vi "test_harness_distance_between_points_squared.vi"() -> ()   [LabVIEW 2009]
panel:
  out "x = y?":bool
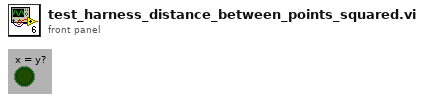
[diagram p1: front panel]
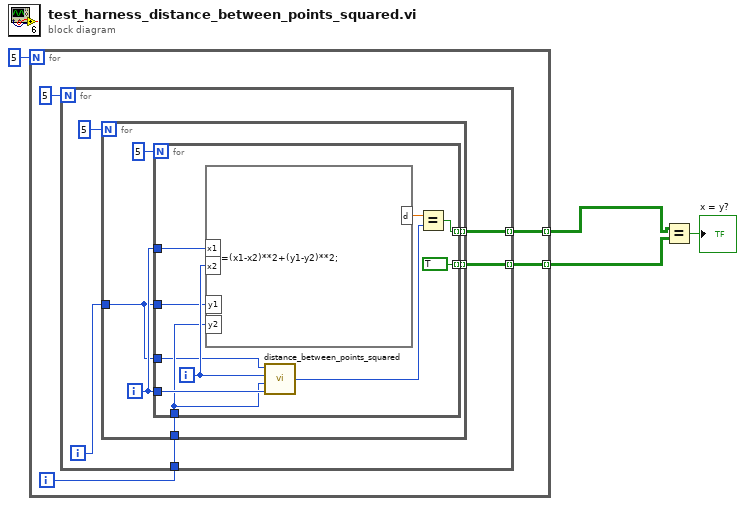
[diagram p0: block diagram]
diagram:
  n1 = for {
    N: 5 -> [_]
    tunnel: [w6] -> w3 mode=indexing
    tunnel: [w5] -> w2 mode=indexing
    i -> [w8]
    n2 = for {
      N: 5 -> [_]
      tunnel: w8 -> [w11]
      tunnel: [w10] -> w6 mode=indexing
      tunnel: [w9] -> w5 mode=indexing
      i -> [w12]
      n3 = for {
        N: 5 -> [_]
        tunnel: w12 -> [w17]
        tunnel: w11 -> [w18]
        tunnel: [w15] -> w10 mode=indexing
        tunnel: [w14] -> w9 mode=indexing
        i -> [w19]
        n4 = for {
          N: 5 -> [_]
          tunnel: w19 -> [w29]
          tunnel: w19 -> [w26]
          tunnel: w17 -> [w24]
          tunnel: w18 -> [w23]
          tunnel: w17 -> [w22]
          tunnel: [w21] -> w15 mode=indexing
          tunnel: [TRUE] -> w14 mode=indexing
          i -> [w25]
          n5 = formula code="d=(x1-x2)**2+(y1-y2)**2;"("x1"=w29, "x2"=w25, "y1"=w24, "y2"=w23) -> ("d"=w27:dbl)
          n6 = call "distance_between_points_squared.vi"("x LIDAR position"=w26, "y LIDAR position"=w23, "x position"=w25, "y position"=w22) -> ("distance squared"=w28:i16)  [unwired: 2 in]
          n7 = Equal?(x=w27, y=w28) -> (x = y?=w21:bool)
        }
      }
    }
  }
  n8 = Equal?(x=w3, y=w2) -> (x = y?=→"x = y?":bool)
